vi "RP Read RX FIFO Fast.vi"(6 "Samples per read":i32=1024, 8 "Error In":errorcluster, 11 "connection ID":refnum<k5>) -> (0 "Error Out":errorcluster, 2 "FIFO out":i32[](array[numeric]), 3 "connection ID out":refnum<k5>)   [LabVIEW 2015]
uses:
  RP Command.ctl
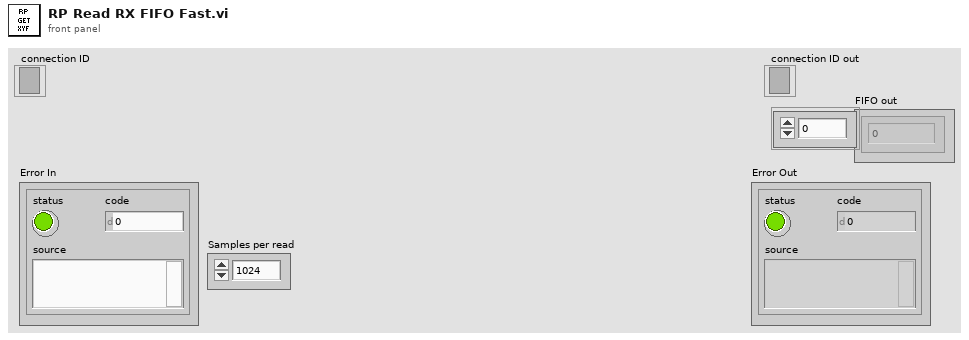
[diagram p1: front panel]
types:
  T1 = enum16{"big-endian, network order", "native, host order", "little-endian"}
  T2 = typedef "RP Command.ctl" = enum16{"Set frequency", "Arm and get data", "Stop server", "Get status", "Get temperature", "Set decimation", "Arm", "Software trigger", "Get whole buffer", "Get chunk", "System call", "Get config", "Set config", "Read FIFO", "Play pattern", "Set frequency batch"}
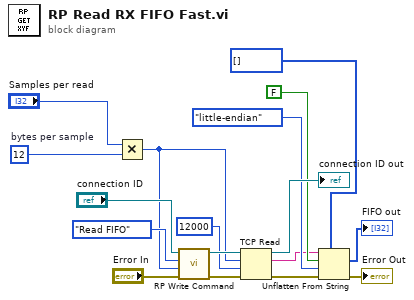
[diagram p0: block diagram]
diagram:
  w3 = 12  # bytes per sample
  n1 = Multiply(x="Samples per read", y=w3) -> (x*y=w1:i32)
  n2 = call "RP Write Command.vi"("Error In"="Error In", "Command payload"=w1, "Command number"=RP_Command."Read FIFO", "connection ID"="connection ID") -> ("Error Out"=w15:errorcluster, "connection ID out"=w16:refnum<k5>)  [unwired: 5 in, 1 out]
  n3 = TCP Read(connection ID=w16, bytes to read=w1, error in (no error)=w15, 9:12000 ("timeout ms (25000)")) -> (connection ID out=→"connection ID out":refnum<k5>, data out=w7:string, error out=w6:errorcluster)  [unwired: 1 in]
  n4 = Unflatten From String(type=i32[] [], binary string=w7, data includes array or string size? (T)=FALSE, byte order (0:big-endian, network order)=T1."little-endian", error in (no error)=w6) -> (value=→"FIFO out":i32[], error out=→"Error Out":errorcluster)  [unwired: 1 out]
